vi "CSM - MassData Update Status Indicator.vi"(8 "error in (no error)":errorcluster, 11 "MassData Status Indicator":refnum<vi>) -> (0 "error out":errorcluster)   [LabVIEW 2017]
uses:
  _support/Operation-FGV-MassData.ctl
  <userlib>/_OpenG.lib/comparison/comparison.llb/I32 Changed__ogtk.vi
  CSM MassData Parameter Support.lvlib
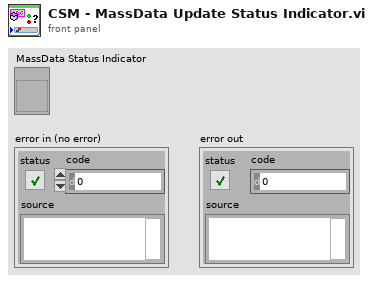
[diagram p1: front panel]
types:
  T1 = typedef "CSM MassData Parameter Support.lvlib/Operation-FGV-MassData.ctl" = enum16{"Initialize", "Read", "Write", "Status", "Release"}
  T2 = typedef "CSM MassData Parameter Support.lvlib/Def-MassDataOper-Status.ctl" = cluster{"Start":i32, "Size":i32, "Total":i32}
  T3 = cluster{cluster{i32, "Start":i32}, cluster{i32, "Start":i32}}
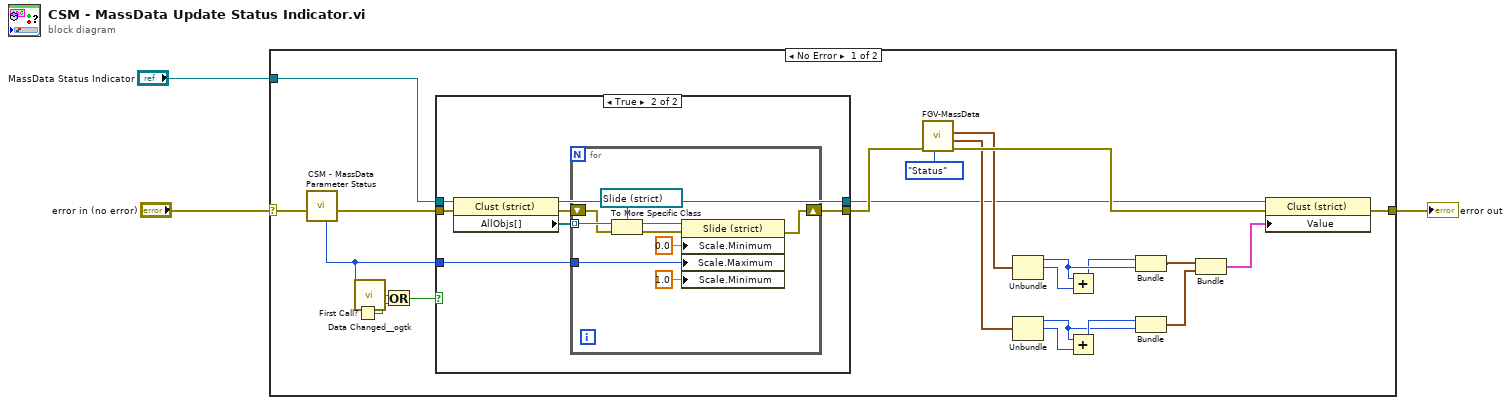
[diagram p0: block diagram]
diagram:
  n1 = case shown="No Error" "error in (no error)" {
    selector: "error in (no error)" -> [w12 w45]
    tunnel: [w26 w45] -> w3
    tunnel: "MassData Status Indicator" -> [w6 _]
    frame No Error {
      n2 = call "CSM - MassData Parameter Status.vi"("Error in"=w12) -> ("Error out"=w11:errorcluster, "cache size"=w9:i32)  [unwired: 6 in, 2 out]
      n3 = First Call?() -> (First Call?: T/F=w7:bool)
      n4 = call-poly <userlib>:"Data Changed__ogtk.vi"("I32"=w9) -> ("Changed"=w8:bool)
      n5 = Or(x=w8, y=w7) -> (x .or. y?=w4:bool)
      n6 = case shown="True" w4 {
        tunnel: w11 -> [w28 w35]
        tunnel: [w28 w32] -> w10
        tunnel: w9 -> [_ w31]
        tunnel: w6 -> [w27 w30]
        tunnel: [w27 w29] -> w5
        frame False {
        }
        frame True {
          n7 = property on="Property Node" class="Clust (strict)"(reference=w30, error in=w35) -> (reference out=w29:refnum<vi>, error out=w33:errorcluster, "AllObjs[]"=w34:refnum<vi>[])
          n8 = for {
            tunnel: w34 -> [w44] mode=indexing
            tunnel: w31 -> [w41]
            shift-right: [w36] -> w32
            shift-left: w33 -> [w38]
            n9 = To More Specific Class(target class=refnum<vi> refnum ("w"), reference=w44, error in=w38) -> (specific class reference=w43:refnum<vi>, error out=w37:errorcluster)
            n10 = property on="Property Node" class="Slide (strict)"(reference=w43, error in=w37, "Scale.Minimum"=0.0 ("Scale.Range:Minimum"), "Scale.Maximum"=w41, "Scale.Minimum"=1.0 ("Scale.Range:Minimum")) -> (error out=w36:errorcluster)  [unwired: 1 out]
          }
        }
      }
      n11 = call "FGV-MassData.vi"("Operation"=Operation-FGV-MassData."Status", "Error in"=w10) -> ("Error out"=w24:errorcluster, "Active Read Oper"=w15:T2, "Active Write Oper"=w19:T2)  [unwired: 6 in, 1 out]
      n12 = Unbundle(w19) -> ("Start"=w22:i32, "Size"=w20:i32)  [unwired: 1 out]
      n13 = Unbundle(w15) -> ("Start"=w16:i32, "Size"=w18:i32)  [unwired: 1 out]
      n14 = Add(x=w22, y=w20) -> (x+y=w21:i32)
      n15 = Add(x=w16, y=w18) -> (x+y=w17:i32)
      n16 = Bundle(w21, "Start"=w22) -> (w14:cluster{i32, "Start":i32})  [unwired: 1 in]
      n17 = Bundle(w17, "Start"=w16) -> (w13:cluster{i32, "Start":i32})  [unwired: 1 in]
      n18 = Bundle(w14, w13) -> (w25:T3)  [unwired: 1 in]
      n19 = property on="Property Node" class="Clust (strict)"(reference=w5, error in=w24, "Value"=w25) -> (error out=w26:errorcluster)  [unwired: 1 out]
    }
    frame Error {
    }
  }
  "error out" <- w3
